vi "Wait For Plugin Response.vi"(8 "error in (no error)":errorcluster, 9 "timeout in ms (0)":i32 format="%d ms", 11 "Plugin Interface in":refnum<class "Plugin Interface.lvclass">) -> (0 "error out":errorcluster, 2 "response":T1, 3 "Plugin Interface out":refnum<class "Plugin Interface.lvclass">, 4 "# elements":u32)   [LabVIEW 2017, in "DSF Core.lvlib" / "Plugin Interface.lvclass"]
uses:
  Plugin Interface.lvclass
  C:/Git/niveristand-data-sharing-framework-custom-device/Core/Classes/Interface/Interface.lvclass
  Response Data.ctl
  Response.ctl
  Response Parameters.ctl
  Dispatcher/Response Timeout.vi
  Interface.lvclass
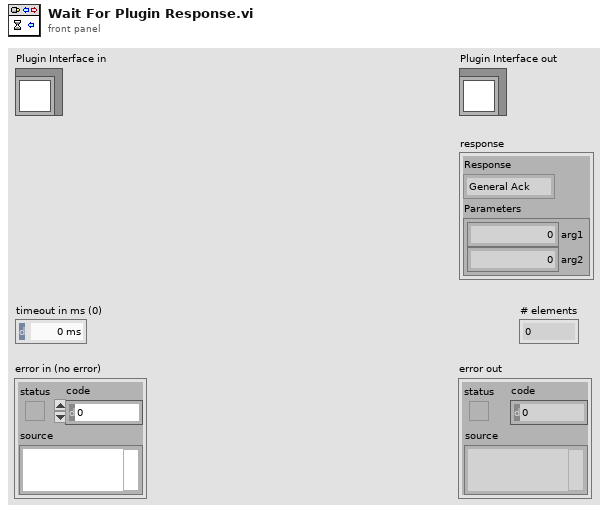
[diagram p1: front panel]
types:
  T1 = typedef "DSF Core.lvlib/Plugin Interface.lvclass/Response Data.ctl" = cluster{"Response":T2, "Parameters":T3}
  T2 = typedef "DSF Core.lvlib/Plugin Interface.lvclass/Response.ctl" = enum8{"General Ack", "Shutting Down"}
  T3 = typedef "DSF Core.lvlib/Plugin Interface.lvclass/Response Parameters.ctl" = cluster{"arg1":u64, "arg2":u64}
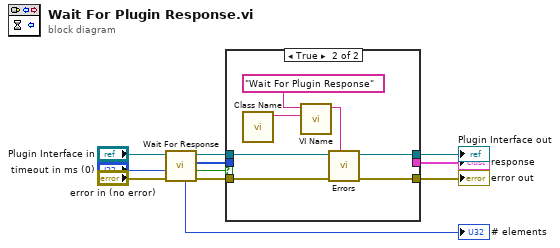
[diagram p0: block diagram]
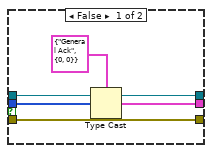
[diagram p2: hidden frame]
diagram:
  n1 = call "Wait For Response.vi"("error in (no error)"="error in (no error)", "timeout in ms (0)"="timeout in ms (0)", "Interface in"="Plugin Interface in") -> ("error out"=w6:errorcluster, "timed out?"=w4:bool, "response data"=w5:u8[], "Interface out"=w7:refnum<class "Plugin Interface.lvclass">, "# elements"=→"# elements":u32)  [unwired: 4 in]
  n2 = case shown="True" w4 {
    tunnel: w6 -> [w15 w23]
    tunnel: w7 -> [w16 w20]
    tunnel: [w16 w22] -> w2
    tunnel: [w15 w21] -> w3
    tunnel: w5 -> [w13 _]
    tunnel: [w14 _] -> w1
    frame False {
      n3 = Type Cast(type=T1 {"Response"=enum."General Ack", "Parameters"={"arg1"=0, "arg2"=0}} ("Plugin Response"), x=w13) -> (*(type *) &x=w14:T1)
    }
    frame True {
      n4 = call "Class Name.vi"() -> ("class name"=w18:string)  [unwired: 11 in]
      n5 = call "VI Name.vi"("class name (\"\")"=w18, "vi name"="Wait For Plugin Response" ("error source vi name")) -> ("full VI name"=w17:string)  [unwired: 9 in]
      n6 = call-poly "Errors.vi"("error source vi name"=w17, "error in (no error)"=w23, "Interface in"=w20) -> ("error out"=w21:errorcluster, "Interface out"=w22:refnum<class "Plugin Interface.lvclass">)  [unwired: 7 in]
    }
  }
  "error out" <- w3
  "Plugin Interface out" <- w2
  "response" <- w1
